vi "VISA speed benchmark.vi"() -> ()   [LabVIEW 2020]
uses:
  Instruments/Vector Network Analyzer/VNA-Keysight PNA/VNA-Keysight PNA.lvclass
  C:/Sandbox/RF Bench/Source Code/WiSpry Test Framework/Instruments/Instrument.lvclass
  C:/Sandbox/RF Bench/Source Code/WiSpry Test Framework/Instruments/Vector Network Analyzer/Vector Network Analyzer.lvclass
  Instruments/Instrument.lvclass/Instrument.ctl
  Instruments/Vector Network Analyzer/Vector Network Analyzer.lvclass/Vector Network Analyzer.ctl
  <instrlib>/Keysight PNA Series/Keysight PNA Series.lvlib
  Instruments/Instrument.lvclass
  Instruments/Vector Network Analyzer/Vector Network Analyzer.lvclass
panel:
  in  "Parameters":cluster{"Name":string, "Value":string}[](array[cluster])
  in  "Path":path
  in  "Save":bool
  out "error out":errorcluster
  out "Sweep Time":dbl
  in  "Test":enum16{"*OPC?", "PNA S-parameters"}(ring)
  out "Average time per query (ms)":dbl
  in  "Repeat":i32=1
  out "read buffer":string
  in  "VISA resource name":refnum<visa-resource-name>
  out "Total time (s)":dbl
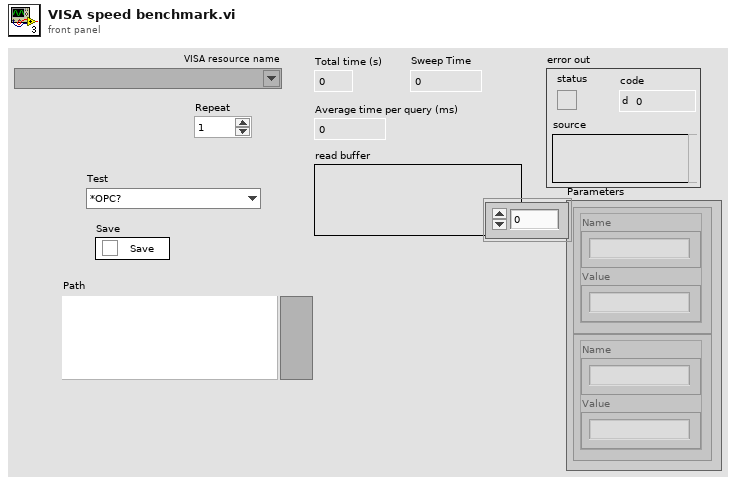
[diagram p1: front panel]
types:
  T1 = typedef "Vector Network Analyzer.lvclass/Sparameter cluster.ctl" = cluster{"Frequency":dbl, "S Parameters":cdb[]}
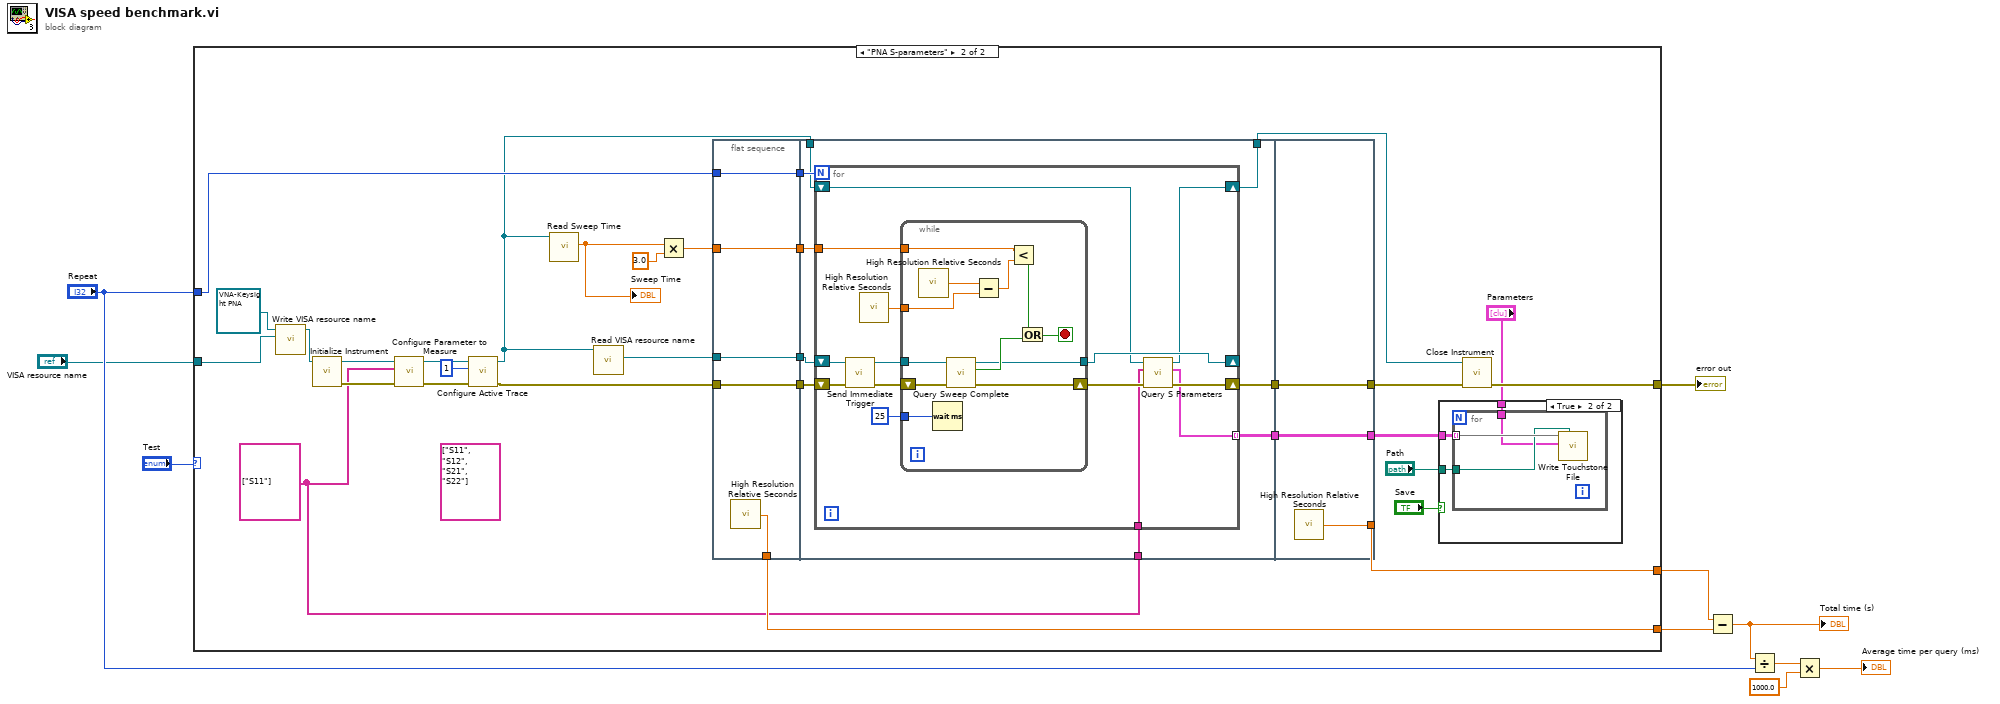
[diagram p0: block diagram]
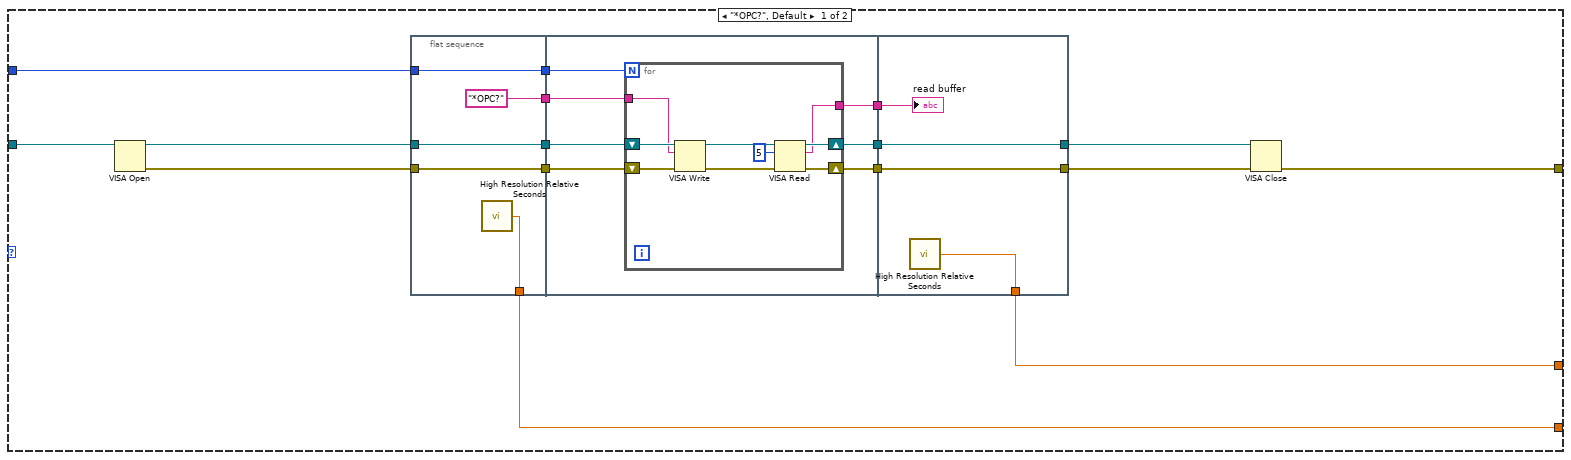
[diagram p2: hidden frame]
diagram:
  n1 = case shown="\"PNA S-parameters\"" "Test" {
    tunnel: [w19 w73] -> w10
    tunnel: [w18 w74] -> w9
    tunnel: "Repeat" -> [w17 w80]
    tunnel: "VISA resource name" -> [w14 w67]
    tunnel: [w11 w61] -> w1
    frame "*OPC?", Default {
      n2 = VISA Open(VISA resource name=w14) -> (VISA resource name=w15:refnum<visa-resource-name>, error out=w16:errorcluster)  [unwired: 4 in]
      n3 = flat-sequence {
        tunnel: w16 -> [w30]
        tunnel: w15 -> [w31]
        tunnel: [w31] -> w26
        tunnel: [w30] -> w25
        tunnel: [w29] -> w19
        tunnel: ["*OPC?" ("write buffer")] -> w24
        tunnel: [w27] -> w23
        tunnel: w17 -> [w27]
        tunnel: w26 -> [w38]
        tunnel: w25 -> [w37]
        tunnel: [w36] -> w22
        tunnel: [w35] -> w21
        tunnel: w24 -> [w34]
        tunnel: [w33] -> w20
        tunnel: w23 -> [w32]
        tunnel: [w50] -> w13
        tunnel: [w51] -> w12
        tunnel: w22 -> [w51]
        tunnel: w21 -> [w50]
        tunnel: [w49] -> w18
        tunnel: w20 -> [w48]
        frame #0 {
          n4 = call <vilib>:"High Resolution Relative Seconds.vi"() -> ("relative seconds"=w29:dbl)
        }
        frame #1 {
          n5 = for {
            N: w32 -> [_]
            tunnel: w34 -> [w41]
            tunnel: [w40] -> w33
            shift-right: [w43] -> w36
            shift-left: w38 -> [w47]
            shift-right: [w42] -> w35
            shift-left: w37 -> [w46]
            n6 = VISA Write(VISA resource name=w47, write buffer=w41, error in (no error)=w46) -> (VISA resource name out=w44:refnum<visa-resource-name>, error out=w45:errorcluster)  [unwired: 1 out]
            n7 = VISA Read(VISA resource name=w44, byte count=u32 5, error in (no error)=w45) -> (VISA resource name out=w43:refnum<visa-resource-name>, read buffer=w40:string, error out=w42:errorcluster)  [unwired: 1 out]
          }
        }
        frame #2 {
          n8 = call <vilib>:"High Resolution Relative Seconds.vi"() -> ("relative seconds"=w49:dbl)
          "read buffer" <- w48
        }
      }
      n9 = VISA Close(VISA resource name=w12, error in (no error)=w13) -> (error out=w11:errorcluster)
    }
    frame "PNA S-parameters" {
      (unwired) string[] ["S11", "S12", "S21", "S22"] ("Sparameters (string)")
      w65 = string[] ["S11"] ("Sparameters (string)")
      n10 = call "Write VISA resource name.vi"("VISA resource name"=w67, "Instrument in"=refnum<class "VNA-Keysight PNA.lvclass"> refnum ("VNA-Keysight PNA.lvclass")) -> ("Instrument out"=w72:refnum<class "VNA-Keysight PNA.lvclass">)  [unwired: 9 in]
      n11 = call-dynamic "Initialize Instrument.vi"("VNA-Keysight PNA in"=w72) -> ("error out"=w66:errorcluster, "VNA-Keysight PNA out"=w68:refnum<class "VNA-Keysight PNA.lvclass">)  [unwired: 9 in]
      n12 = call-dynamic "Configure Parameter to Measure.vi"("error in (no error)"=w66, "Sparameters (string)"=w65, "VNA-Keysight PNA in"=w68) -> ("error out"=w71:errorcluster, "VNA-Keysight PNA out"=w70:refnum<class "VNA-Keysight PNA.lvclass">)  [unwired: 7 in]
      n13 = call-dynamic "Configure Active Trace.vi"("error in (no error)"=w71, "Active Trace"=u8 1, "VNA-Keysight PNA in"=w70) -> ("error out"=w64:errorcluster, "VNA-Keysight PNA out"=w60:refnum<class "VNA-Keysight PNA.lvclass">)  [unwired: 7 in]
      n14 = call "Read Sweep Time.vi"("Vector Network Analyzer in"=w60) -> ("Sweep Time"=w59:dbl)  [unwired: 9 in, 1 out]
      "Sweep Time" <- w59
      n15 = call "Read VISA resource name.vi"("Instrument in"=w60) -> ("VISA resource name"=w63:refnum<visa-resource-name>)  [unwired: 9 in, 1 out]
      n16 = Multiply(x=w59, y=3.0) -> (x*y=w81:dbl)
      n17 = flat-sequence {
        tunnel: w80 -> [w90]
        tunnel: w63 -> [w91]
        tunnel: w64 -> [w92]
        tunnel: w81 -> [w93]
        tunnel: [w93] -> w78
        tunnel: [w92] -> w77
        tunnel: [w91] -> w76
        tunnel: [w90] -> w75
        tunnel: [w89] -> w73
        tunnel: w60 -> [w95]
        tunnel: [w100] -> w79
        tunnel: w78 -> [w102]
        tunnel: w77 -> [w101]
        tunnel: w76 -> [w99]
        tunnel: w75 -> [w98]
        tunnel: w65 -> [w97]
        tunnel: [w96] -> w58
        tunnel: [w94] -> w56
        tunnel: [w131] -> w62
        tunnel: w79 -> [w131]
        tunnel: [w130] -> w74
        tunnel: w56 -> [w129]
        tunnel: [w129] -> w55
        frame #0 {
          n18 = call <vilib>:"High Resolution Relative Seconds.vi"() -> ("relative seconds"=w89:dbl)
        }
        frame #1 {
          n19 = for {
            N: w98 -> [_]
            tunnel: w102 -> [w112]
            shift-right: [w109] -> w100
            shift-left: w101 -> [w111]
            shift-right: [w107] -> _
            shift-left: w99 -> [w108]
            tunnel: w97 -> [w106]
            shift-right: [w105] -> w96
            shift-left: w95 -> [w104]
            tunnel: [w103] -> w94 mode=indexing
            n20 = call <instrlib>:"Send Immediate Trigger.vi"("error in (no error)"=w111, "VISA resource name"=w108) -> ("error out"=w116:errorcluster, "VISA resource name out"=w115:refnum<visa-resource-name>)  [unwired: 8 in]
            n21 = call <vilib>:"High Resolution Relative Seconds.vi"() -> ("relative seconds"=w113:dbl)
            n22 = while {
              tunnel: w115 -> [w126]
              shift-right: [w127] -> w110
              shift-left: w116 -> [w128]
              tunnel: u32 25 ("milliseconds to wait") -> [w125]
              tunnel: w113 -> [w124]
              tunnel: w112 -> [w121]
              tunnel: [w117] -> w107
              stop <- w118 stop-if-true
              n23 = call <vilib>:"High Resolution Relative Seconds.vi"() -> ("relative seconds"=w123:dbl)
              n24 = Wait (ms)(milliseconds to wait=w125) -> ()  [unwired: 1 out]
              n25 = call <instrlib>:"Query Sweep Complete.vi"("error in (no error)"=w128, "VISA resource name"=w126) -> ("error out"=w127:errorcluster, "Sweep Complete"=w122:bool, "VISA resource name out"=w117:refnum<visa-resource-name>)  [unwired: 7 in]
              n26 = Subtract(x=w123, y=w124) -> (x-y=w120:dbl)
              n27 = Less?(x=w121, y=w120) -> (x < y?=w119:bool)
              n28 = Or(x=w119, y=w122) -> (x .or. y?=w118:bool)
            }
            n29 = call-dynamic "Query S Parameters.vi"("error in (no error)"=w110, "Sparameters (string)"=w106, "VNA-Keysight PNA in"=w104) -> ("error out"=w109:errorcluster, "S parameters"=w103:T1[], "VNA-Keysight PNA out"=w105:refnum<class "VNA-Keysight PNA.lvclass">)  [unwired: 6 in]
          }
        }
        frame #2 {
          n30 = call <vilib>:"High Resolution Relative Seconds.vi"() -> ("relative seconds"=w130:dbl)
        }
      }
      n31 = case shown="True" "Save" {
        tunnel: w55 -> [_ w85]
        tunnel: "Path" -> [_ w84]
        tunnel: "Parameters" -> [_ w83]
        frame False {
        }
        frame True {
          n32 = for {
            tunnel: w85 -> [w88] mode=indexing
            tunnel: w84 -> [w87]
            tunnel: w83 -> [w86]
            n33 = call "Write Touchstone File.vi"("File Path"=w87, "Parameters"=w86, "Sparameters"=w88) -> ()  [unwired: 8 in, 1 out]
          }
        }
      }
      n34 = call-dynamic "Close Instrument.vi"("error in (no error)"=w62, "VNA-Keysight PNA in"=w58) -> ("error out"=w61:errorcluster)  [unwired: 8 in, 1 out]
    }
  }
  "error out" <- w1
  n35 = Subtract(x=w9, y=w10) -> (x-y=w8:dbl)
  "Total time (s)" <- w8
  n36 = Divide(x=w8, y="Repeat") -> (x/y=w5:dbl)
  n37 = Multiply(x=w5, y=1000.0) -> (x*y=→"Average time per query (ms)":dbl)
